vi "_r2aio_16bit_8in_canopen_master.vi"() -> ()   [LabVIEW 2011]
panel:
  out "ret write_device_object_sdo INT":i16
  out "ret write_pdo_mapping 12":i16
  out "Analogue IN 8":i16
  out "ret read_node_object_dictionary 8":i16
  out "Analogue IN 7":i16
  out "ret read_node_object_dictionary 7":i16
  out "Analogue IN 6":i16
  out "ret read_node_object_dictionary 6":i16
  out "Analogue IN 5":i16
  out "ret read_node_object_dictionary 5":i16
  out "Analogue IN 4":i16
  out "ret read_node_object_dictionary 4":i16
  out "Analogue IN 3":i16
  out "ret read_node_object_dictionary 3":i16
  out "Analogue IN 2":i16
  out "ret read_node_object_dictionary 2":i16
  out "Analogue IN 1":i16
  out "ret write_pdo_mapping 11":i16
  out "ret write_pdo_mapping 10":i16
  out "ret write_pdo_mapping 9":i16
  out "ret write_pdo_mapping 8":i16
  out "ret write_pdo_mapping 7":i16
  out "ret write_pdo_mapping 6":i16
  out "ret write_pdo_mapping 5":i16
  out "ret write_pdo_mapping 4":i16
  out "ret write_pdo_mapping 2":i16
  out "ret add_node_object_dictionary 6401-8":i16
  out "ret add_node_object_dictionary 6401-7":i16
  out "ret add_node_object_dictionary 6401-6":i16
  out "ret add_node_object_dictionary 6401-5":i16
  out "ret add_node_object_dictionary 6401-4":i16
  out "ret add_node_object_dictionary 6401-3":i16
  out "ret add_node_object_dictionary 6401-2":i16
  out "datasize":u32
  out "Manufacturer software ver":string
  out "ret read_device_object_sdo 3":i16
  out "datasize":u32
  out "Manufacturer hardware ver":string
  out "ret read_device_object_sdo 2":i16
  out "datasize":u32
  out "Manufacturer dev name":string
  out "ret read_device_object_sdo 1":i16
  out "ret read_node_object_dictionary 1":i16
  in  "stop monitor":bool
  out "ret write_master_hbt":i16
  out "ret stop_can_master":i16
  out "ret write_pdo_mapping 3":i16
  out "ret write_pdo_mapping 1":i16
  out "ret add_node_object_dictionary 6401-1":i16
  out "ret write_device_object_sdo HBT":i16
  in  "slave node":u8
  in  "baudrate":T1(ring)
  in  "net":u8
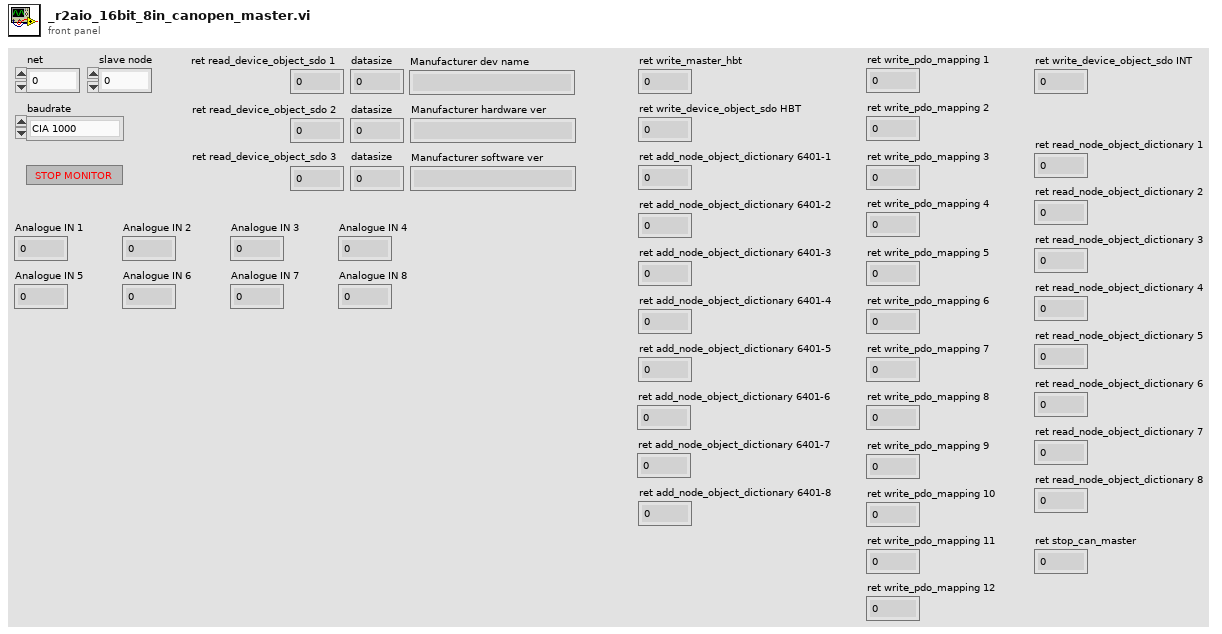
[diagram p1: front panel]
types:
  T1 = enum8{"CIA 1000", "CIA 800", "CIA 500", "CIA 250", "CIA 125", "CIA 100", "CIA 50", "CIA 20", "CIA 10", "CIA AUTO"}
diagram:
  n1 = flat-sequence {
    tunnel: ["slave node"] -> w44
    tunnel: w44 -> [w54]
    tunnel: [w54] -> w43
    tunnel: w43 -> [w56]
    tunnel: [w56] -> w46
    tunnel: w46 -> [w63]
    tunnel: [w63] -> w45
    tunnel: w45 -> [w66]
    tunnel: [w66] -> w40
    tunnel: w40 -> [w71]
    tunnel: [w71] -> w39
    tunnel: w39 -> [w76]
    tunnel: [w76] -> w38
    tunnel: w38 -> [w81]
    tunnel: [w81] -> w37
    tunnel: w37 -> [w86]
    tunnel: [w86] -> w36
    tunnel: w36 -> [w91]
    tunnel: [w91] -> w35
    tunnel: w35 -> [w97]
    tunnel: [w97] -> w34
    tunnel: w34 -> [w101]
    tunnel: [w101] -> w9
    tunnel: [w106] -> w42
    tunnel: w9 -> [w106]
    tunnel: [w111] -> w33
    tunnel: w42 -> [w111]
    tunnel: [w108] -> w21
    tunnel: w33 -> [w121]
    tunnel: [w121] -> w22
    tunnel: w21 -> [w119]
    tunnel: [w119] -> w20
    tunnel: [w128] -> w32
    tunnel: [w126] -> w19
    tunnel: w22 -> [w128]
    tunnel: w20 -> [w126]
    tunnel: w32 -> [w135]
    tunnel: [w135] -> w31
    tunnel: w19 -> [w133]
    tunnel: [w133] -> w18
    tunnel: w31 -> [w141]
    tunnel: [w141] -> w30
    tunnel: w18 -> [w140]
    tunnel: [w140] -> w17
    tunnel: w30 -> [w149]
    tunnel: [w149] -> w29
    tunnel: w17 -> [w147]
    tunnel: [w147] -> w16
    tunnel: w29 -> [w155]
    tunnel: [w155] -> w28
    tunnel: w16 -> [w154]
    tunnel: [w154] -> w15
    tunnel: w28 -> [w163]
    tunnel: [w163] -> w27
    tunnel: w15 -> [w161]
    tunnel: [w161] -> w14
    tunnel: w27 -> [w169]
    tunnel: [w169] -> w26
    tunnel: w14 -> [w168]
    tunnel: [w168] -> w13
    tunnel: w26 -> [w176]
    tunnel: [w176] -> w25
    tunnel: w13 -> [w175]
    tunnel: [w175] -> w12
    tunnel: [w184] -> w24
    tunnel: [w182] -> w11
    tunnel: w12 -> [w182]
    tunnel: w25 -> [w184]
    tunnel: w24 -> [w191]
    tunnel: [w191] -> w23
    tunnel: w11 -> [w189]
    tunnel: [w189] -> w10
    tunnel: [w202] -> w41
    tunnel: w10 -> [_]
    tunnel: w23 -> [w202]
    tunnel: [w204] -> w5
    tunnel: w41 -> [w204]
    tunnel: [w212] -> w7
    tunnel: w5 -> [w212]
    tunnel: w7 -> [w214]
    tunnel: [w214] -> w6
    tunnel: w6 -> [w215]
    tunnel: [w215] -> w4
    tunnel: w4 -> [w224]
    tunnel: [w224] -> w3
    tunnel: w3 -> [w225]
    tunnel: [w225] -> w2
    tunnel: w2 -> [w234]
    tunnel: [w234] -> w1
    tunnel: w1 -> [w236]
    tunnel: [w236] -> w8
    tunnel: w8 -> [w237]
    frame #0 {
      # "Start CAN master"
      n2 = call "start_can_master.vi"("br"="baudrate", "net"="net") -> ("return"=w50:i16)  [unwired: 9 in]
      n3 = Not Equal To 0?(x=w50) -> (x != 0?=w49:bool)
      n4 = Stop(stop? (T)=w49) -> ()
    }
    frame #1 {
      w52 = u8 129 items=["CAN_NMT_CS_DUMMY"=0, "CAN_NMT_START_REMOTE_NODE"=1, "CAN_NMT_STOP_REMOTE_NODE"=2, "CAN_NMT_ENTER_PRE_OPERATIONAL"=128, "CAN_NMT_RESET_NODE"=129, "CAN_NMT_RESET_COMMUNICATION"=130]  # NMT spec
      # "NMT Reset node"
      n5 = call "nmt_master_command.vi"("node"="slave node", "cs"=w52) -> ()  [unwired: 10 in]
    }
    frame #2 {
      n6 = Wait (ms)(milliseconds to wait=u32 500) -> ()  [unwired: 1 out]
    }
    frame #3 {
      # "Configure MASTER Heartbeat"
      n7 = call "write_master_hbt.vi"("hbt"=u16 1200, "node"=w56) -> ("return"=→"ret write_master_hbt":i16)  [unwired: 9 in]
    }
    frame #4 {
      # "Configure SLAVE Heartbeat"
      n8 = Build Array(u8 232, u8 3) -> (w59:u8[])
      n9 = call "write_device_object_sdo.vi"("node"=w63, "index"=u16 4119, "subind"=u8 0, "data"=w59, "datasize"=u32 2) -> ("return"=→"ret write_device_object_sdo HBT":i16)  [unwired: 10 in]
    }
    frame #5 {
      w68 = u16 3 items=["CAN_DEFTYPE_BOOLEAN"=1, "CAN_DEFTYPE_INTEGER8"=2, "CAN_DEFTYPE_INTEGER16"=3, "CAN_DEFTYPE_INTEGER32"=4, "CAN_DEFTYPE_UNSIGNED8"=5, "CAN_DEFTYPE_UNSIGNED16"=6, "CAN_DEFTYPE_UNSIGNED32"=7, "CAN_DEFTYPE_REAL32"=8, "CAN_DEFTYPE_VISIBLE_STRING"=9, "CAN_DEFTYPE_OCTET_STRING"=10, "CAN_DEFTYPE_UNICODE_STRING"=11, "CAN_DEFTYPE_TIME_OF_DAY"=12, "CAN_DEFTYPE_TIME_DIFFERENCE"=13, "CAN_DEFTYPE_DOMAIN"=15, "CAN_DEFTYPE_INTEGER24"=16, "CAN_DEFTYPE_REAL64"=17, "CAN_DEFTYPE_INTEGER40"=18, "CAN_DEFTYPE_INTEGER48"=19, "CAN_DEFTYPE_INTEGER56"=20, "CAN_DEFTYPE_INTEGER64"=21, "CAN_DEFTYPE_UNSIGNED24"=22, "CAN_DEFTYPE_UNSIGNED40"=24, "CAN_DEFTYPE_UNSIGNED48"=25, "CAN_DEFTYPE_UNSIGNED56"=26, "CAN_DEFTYPE_UNSIGNED64"=27]  # Data type spec
      # "Add Read Analogue input 1 object to MASTER dictionary"
      n10 = call "add_node_object_dictionary.vi"("type"=w68, "subind"=u8 1, "index"=u16 25601, "node"=w66) -> ("return"=→"ret add_node_object_dictionary 6401-1":i16)  [unwired: 7 in]
    }
    frame #6 {
      w73 = u16 3 items=["CAN_DEFTYPE_BOOLEAN"=1, "CAN_DEFTYPE_INTEGER8"=2, "CAN_DEFTYPE_INTEGER16"=3, "CAN_DEFTYPE_INTEGER32"=4, "CAN_DEFTYPE_UNSIGNED8"=5, "CAN_DEFTYPE_UNSIGNED16"=6, "CAN_DEFTYPE_UNSIGNED32"=7, "CAN_DEFTYPE_REAL32"=8, "CAN_DEFTYPE_VISIBLE_STRING"=9, "CAN_DEFTYPE_OCTET_STRING"=10, "CAN_DEFTYPE_UNICODE_STRING"=11, "CAN_DEFTYPE_TIME_OF_DAY"=12, "CAN_DEFTYPE_TIME_DIFFERENCE"=13, "CAN_DEFTYPE_DOMAIN"=15, "CAN_DEFTYPE_INTEGER24"=16, "CAN_DEFTYPE_REAL64"=17, "CAN_DEFTYPE_INTEGER40"=18, "CAN_DEFTYPE_INTEGER48"=19, "CAN_DEFTYPE_INTEGER56"=20, "CAN_DEFTYPE_INTEGER64"=21, "CAN_DEFTYPE_UNSIGNED24"=22, "CAN_DEFTYPE_UNSIGNED40"=24, "CAN_DEFTYPE_UNSIGNED48"=25, "CAN_DEFTYPE_UNSIGNED56"=26, "CAN_DEFTYPE_UNSIGNED64"=27]  # Data type spec
      # "Add Read Analogue input 2 object to MASTER dictionary"
      n11 = call "add_node_object_dictionary.vi"("type"=w73, "subind"=u8 2, "index"=u16 25601, "node"=w71) -> ("return"=→"ret add_node_object_dictionary 6401-2":i16)  [unwired: 7 in]
    }
    frame #7 {
      w78 = u16 3 items=["CAN_DEFTYPE_BOOLEAN"=1, "CAN_DEFTYPE_INTEGER8"=2, "CAN_DEFTYPE_INTEGER16"=3, "CAN_DEFTYPE_INTEGER32"=4, "CAN_DEFTYPE_UNSIGNED8"=5, "CAN_DEFTYPE_UNSIGNED16"=6, "CAN_DEFTYPE_UNSIGNED32"=7, "CAN_DEFTYPE_REAL32"=8, "CAN_DEFTYPE_VISIBLE_STRING"=9, "CAN_DEFTYPE_OCTET_STRING"=10, "CAN_DEFTYPE_UNICODE_STRING"=11, "CAN_DEFTYPE_TIME_OF_DAY"=12, "CAN_DEFTYPE_TIME_DIFFERENCE"=13, "CAN_DEFTYPE_DOMAIN"=15, "CAN_DEFTYPE_INTEGER24"=16, "CAN_DEFTYPE_REAL64"=17, "CAN_DEFTYPE_INTEGER40"=18, "CAN_DEFTYPE_INTEGER48"=19, "CAN_DEFTYPE_INTEGER56"=20, "CAN_DEFTYPE_INTEGER64"=21, "CAN_DEFTYPE_UNSIGNED24"=22, "CAN_DEFTYPE_UNSIGNED40"=24, "CAN_DEFTYPE_UNSIGNED48"=25, "CAN_DEFTYPE_UNSIGNED56"=26, "CAN_DEFTYPE_UNSIGNED64"=27]  # Data type spec
      # "Add Read Analogue input 3 object to MASTER dictionary"
      n12 = call "add_node_object_dictionary.vi"("type"=w78, "subind"=u8 3, "index"=u16 25601, "node"=w76) -> ("return"=→"ret add_node_object_dictionary 6401-3":i16)  [unwired: 7 in]
    }
    frame #8 {
      w83 = u16 3 items=["CAN_DEFTYPE_BOOLEAN"=1, "CAN_DEFTYPE_INTEGER8"=2, "CAN_DEFTYPE_INTEGER16"=3, "CAN_DEFTYPE_INTEGER32"=4, "CAN_DEFTYPE_UNSIGNED8"=5, "CAN_DEFTYPE_UNSIGNED16"=6, "CAN_DEFTYPE_UNSIGNED32"=7, "CAN_DEFTYPE_REAL32"=8, "CAN_DEFTYPE_VISIBLE_STRING"=9, "CAN_DEFTYPE_OCTET_STRING"=10, "CAN_DEFTYPE_UNICODE_STRING"=11, "CAN_DEFTYPE_TIME_OF_DAY"=12, "CAN_DEFTYPE_TIME_DIFFERENCE"=13, "CAN_DEFTYPE_DOMAIN"=15, "CAN_DEFTYPE_INTEGER24"=16, "CAN_DEFTYPE_REAL64"=17, "CAN_DEFTYPE_INTEGER40"=18, "CAN_DEFTYPE_INTEGER48"=19, "CAN_DEFTYPE_INTEGER56"=20, "CAN_DEFTYPE_INTEGER64"=21, "CAN_DEFTYPE_UNSIGNED24"=22, "CAN_DEFTYPE_UNSIGNED40"=24, "CAN_DEFTYPE_UNSIGNED48"=25, "CAN_DEFTYPE_UNSIGNED56"=26, "CAN_DEFTYPE_UNSIGNED64"=27]  # Data type spec
      # "Add Read Analogue input 4 object to MASTER dictionary"
      n13 = call "add_node_object_dictionary.vi"("type"=w83, "subind"=u8 4, "index"=u16 25601, "node"=w81) -> ("return"=→"ret add_node_object_dictionary 6401-4":i16)  [unwired: 7 in]
    }
    frame #9 {
      w88 = u16 3 items=["CAN_DEFTYPE_BOOLEAN"=1, "CAN_DEFTYPE_INTEGER8"=2, "CAN_DEFTYPE_INTEGER16"=3, "CAN_DEFTYPE_INTEGER32"=4, "CAN_DEFTYPE_UNSIGNED8"=5, "CAN_DEFTYPE_UNSIGNED16"=6, "CAN_DEFTYPE_UNSIGNED32"=7, "CAN_DEFTYPE_REAL32"=8, "CAN_DEFTYPE_VISIBLE_STRING"=9, "CAN_DEFTYPE_OCTET_STRING"=10, "CAN_DEFTYPE_UNICODE_STRING"=11, "CAN_DEFTYPE_TIME_OF_DAY"=12, "CAN_DEFTYPE_TIME_DIFFERENCE"=13, "CAN_DEFTYPE_DOMAIN"=15, "CAN_DEFTYPE_INTEGER24"=16, "CAN_DEFTYPE_REAL64"=17, "CAN_DEFTYPE_INTEGER40"=18, "CAN_DEFTYPE_INTEGER48"=19, "CAN_DEFTYPE_INTEGER56"=20, "CAN_DEFTYPE_INTEGER64"=21, "CAN_DEFTYPE_UNSIGNED24"=22, "CAN_DEFTYPE_UNSIGNED40"=24, "CAN_DEFTYPE_UNSIGNED48"=25, "CAN_DEFTYPE_UNSIGNED56"=26, "CAN_DEFTYPE_UNSIGNED64"=27]  # Data type spec
      # "Add Read Analogue input 5 object to MASTER dictionary"
      n14 = call "add_node_object_dictionary.vi"("type"=w88, "subind"=u8 5, "index"=u16 25601, "node"=w86) -> ("return"=→"ret add_node_object_dictionary 6401-5":i16)  [unwired: 7 in]
    }
    frame #10 {
      w93 = u16 3 items=["CAN_DEFTYPE_BOOLEAN"=1, "CAN_DEFTYPE_INTEGER8"=2, "CAN_DEFTYPE_INTEGER16"=3, "CAN_DEFTYPE_INTEGER32"=4, "CAN_DEFTYPE_UNSIGNED8"=5, "CAN_DEFTYPE_UNSIGNED16"=6, "CAN_DEFTYPE_UNSIGNED32"=7, "CAN_DEFTYPE_REAL32"=8, "CAN_DEFTYPE_VISIBLE_STRING"=9, "CAN_DEFTYPE_OCTET_STRING"=10, "CAN_DEFTYPE_UNICODE_STRING"=11, "CAN_DEFTYPE_TIME_OF_DAY"=12, "CAN_DEFTYPE_TIME_DIFFERENCE"=13, "CAN_DEFTYPE_DOMAIN"=15, "CAN_DEFTYPE_INTEGER24"=16, "CAN_DEFTYPE_REAL64"=17, "CAN_DEFTYPE_INTEGER40"=18, "CAN_DEFTYPE_INTEGER48"=19, "CAN_DEFTYPE_INTEGER56"=20, "CAN_DEFTYPE_INTEGER64"=21, "CAN_DEFTYPE_UNSIGNED24"=22, "CAN_DEFTYPE_UNSIGNED40"=24, "CAN_DEFTYPE_UNSIGNED48"=25, "CAN_DEFTYPE_UNSIGNED56"=26, "CAN_DEFTYPE_UNSIGNED64"=27]  # Data type spec
      # "Add Read Analogue input 6 object to MASTER dictionary"
      n15 = call "add_node_object_dictionary.vi"("type"=w93, "subind"=u8 6, "index"=u16 25601, "node"=w91) -> ("return"=→"ret add_node_object_dictionary 6401-6":i16)  [unwired: 7 in]
    }
    frame #11 {
      w96 = u16 3 items=["CAN_DEFTYPE_BOOLEAN"=1, "CAN_DEFTYPE_INTEGER8"=2, "CAN_DEFTYPE_INTEGER16"=3, "CAN_DEFTYPE_INTEGER32"=4, "CAN_DEFTYPE_UNSIGNED8"=5, "CAN_DEFTYPE_UNSIGNED16"=6, "CAN_DEFTYPE_UNSIGNED32"=7, "CAN_DEFTYPE_REAL32"=8, "CAN_DEFTYPE_VISIBLE_STRING"=9, "CAN_DEFTYPE_OCTET_STRING"=10, "CAN_DEFTYPE_UNICODE_STRING"=11, "CAN_DEFTYPE_TIME_OF_DAY"=12, "CAN_DEFTYPE_TIME_DIFFERENCE"=13, "CAN_DEFTYPE_DOMAIN"=15, "CAN_DEFTYPE_INTEGER24"=16, "CAN_DEFTYPE_REAL64"=17, "CAN_DEFTYPE_INTEGER40"=18, "CAN_DEFTYPE_INTEGER48"=19, "CAN_DEFTYPE_INTEGER56"=20, "CAN_DEFTYPE_INTEGER64"=21, "CAN_DEFTYPE_UNSIGNED24"=22, "CAN_DEFTYPE_UNSIGNED40"=24, "CAN_DEFTYPE_UNSIGNED48"=25, "CAN_DEFTYPE_UNSIGNED56"=26, "CAN_DEFTYPE_UNSIGNED64"=27]  # Data type spec
      # "Add Read Analogue input 7 object to MASTER dictionary"
      n16 = call "add_node_object_dictionary.vi"("type"=w96, "subind"=u8 7, "index"=u16 25601, "node"=w97) -> ("return"=→"ret add_node_object_dictionary 6401-7":i16)  [unwired: 7 in]
    }
    frame #12 {
      w103 = u16 3 items=["CAN_DEFTYPE_BOOLEAN"=1, "CAN_DEFTYPE_INTEGER8"=2, "CAN_DEFTYPE_INTEGER16"=3, "CAN_DEFTYPE_INTEGER32"=4, "CAN_DEFTYPE_UNSIGNED8"=5, "CAN_DEFTYPE_UNSIGNED16"=6, "CAN_DEFTYPE_UNSIGNED32"=7, "CAN_DEFTYPE_REAL32"=8, "CAN_DEFTYPE_VISIBLE_STRING"=9, "CAN_DEFTYPE_OCTET_STRING"=10, "CAN_DEFTYPE_UNICODE_STRING"=11, "CAN_DEFTYPE_TIME_OF_DAY"=12, "CAN_DEFTYPE_TIME_DIFFERENCE"=13, "CAN_DEFTYPE_DOMAIN"=15, "CAN_DEFTYPE_INTEGER24"=16, "CAN_DEFTYPE_REAL64"=17, "CAN_DEFTYPE_INTEGER40"=18, "CAN_DEFTYPE_INTEGER48"=19, "CAN_DEFTYPE_INTEGER56"=20, "CAN_DEFTYPE_INTEGER64"=21, "CAN_DEFTYPE_UNSIGNED24"=22, "CAN_DEFTYPE_UNSIGNED40"=24, "CAN_DEFTYPE_UNSIGNED48"=25, "CAN_DEFTYPE_UNSIGNED56"=26, "CAN_DEFTYPE_UNSIGNED64"=27]  # Data type spec
      # "Add Read Analogue input 8 object to MASTER dictionary"
      n17 = call "add_node_object_dictionary.vi"("type"=w103, "subind"=u8 8, "index"=u16 25601, "node"=w101) -> ("return"=→"ret add_node_object_dictionary 6401-8":i16)  [unwired: 7 in]
    }
    frame #13 {
      w107 = u8 1 items=["CAN_NMT_CS_DUMMY"=0, "CAN_NMT_START_REMOTE_NODE"=1, "CAN_NMT_STOP_REMOTE_NODE"=2, "CAN_NMT_ENTER_PRE_OPERATIONAL"=128, "CAN_NMT_RESET_NODE"=129, "CAN_NMT_RESET_COMMUNICATION"=130]  # NMT spec
      # "NMT Start remote node"
      n18 = call "nmt_master_command.vi"("node"=w106, "cs"=w107) -> ()  [unwired: 10 in]
    }
    frame #14 {
      # "Disable RPDO2 mapping"
      n19 = Subtract(x=w111, y=u8 1) -> (x-y=w110:u8)
      n20 = Multiply(x=w110, y=u8 4) -> (x*y=w109:u8)
      n21 = To Unsigned Word Integer(number=w109) -> (unsigned 16bit integer=w108:u16)
      n22 = Add(x=w108, y=u16 5633) -> (x+y=w114:u16)
      n23 = call "write_pdo_mapping.vi"("data"=u32 0, "subind"=u8 0, "index"=w114) -> ("return"=→"ret write_pdo_mapping 1":i16)  [unwired: 8 in]
    }
    frame #15 {
      # "Disable RPDO3 mapping"
      n24 = Add(x=w119, y=u16 5634) -> (x+y=w120:u16)
      n25 = call "write_pdo_mapping.vi"("data"=u32 0, "subind"=u8 0, "index"=w120) -> ("return"=→"ret write_pdo_mapping 2":i16)  [unwired: 8 in]
    }
    frame #16 {
      # "Map Read Analogue Input 1 RPDO2"
      n26 = Add(x=w126, y=u16 5633) -> (x+y=w127:u16)
      n27 = call "write_pdo_mapping.vi"("data"=u32 1677787408, "subind"=u8 1, "index"=w127) -> ("return"=→"ret write_pdo_mapping 3":i16)  [unwired: 8 in]
    }
    frame #17 {
      # "Map Read Analogue Input 2 RPDO2"
      n28 = Add(x=w133, y=u16 5633) -> (x+y=w134:u16)
      n29 = call "write_pdo_mapping.vi"("data"=u32 1677787664, "subind"=u8 2, "index"=w134) -> ("return"=→"ret write_pdo_mapping 4":i16)  [unwired: 8 in]
    }
    frame #18 {
      # "Map Read Analogue Input 3 RPDO2"
      n30 = Add(x=w140, y=u16 5633) -> (x+y=w143:u16)
      n31 = call "write_pdo_mapping.vi"("data"=u32 1677787920, "subind"=u8 3, "index"=w143) -> ("return"=→"ret write_pdo_mapping 5":i16)  [unwired: 8 in]
    }
    frame #19 {
      # "Map Read Analogue Input 4 RPDO2"
      n32 = Add(x=w147, y=u16 5633) -> (x+y=w148:u16)
      n33 = call "write_pdo_mapping.vi"("data"=u32 1677788176, "subind"=u8 4, "index"=w148) -> ("return"=→"ret write_pdo_mapping 6":i16)  [unwired: 8 in]
    }
    frame #20 {
      # "Map Read Analogue Input 5 RPDO3"
      n34 = Add(x=w154, y=u16 5634) -> (x+y=w156:u16)
      n35 = call "write_pdo_mapping.vi"("data"=u32 1677788432, "subind"=u8 1, "index"=w156) -> ("return"=→"ret write_pdo_mapping 7":i16)  [unwired: 8 in]
    }
    frame #21 {
      # "Map Read Analogue Input 6 RPDO3"
      n36 = Add(x=w161, y=u16 5634) -> (x+y=w162:u16)
      n37 = call "write_pdo_mapping.vi"("data"=u32 1677788688, "subind"=u8 2, "index"=w162) -> ("return"=→"ret write_pdo_mapping 8":i16)  [unwired: 8 in]
    }
    frame #22 {
      # "Map Read Analogue Input 7 RPDO3"
      n38 = Add(x=w168, y=u16 5634) -> (x+y=w171:u16)
      n39 = call "write_pdo_mapping.vi"("data"=u32 1677788944, "subind"=u8 3, "index"=w171) -> ("return"=→"ret write_pdo_mapping 9":i16)  [unwired: 8 in]
    }
    frame #23 {
      # "Map Read Analogue Input 8 RPDO3"
      n40 = Add(x=w175, y=u16 5634) -> (x+y=w178:u16)
      n41 = call "write_pdo_mapping.vi"("data"=u32 1677789200, "subind"=u8 4, "index"=w178) -> ("return"=→"ret write_pdo_mapping 10":i16)  [unwired: 8 in]
    }
    frame #24 {
      # "Enable RPDO2 mapping"
      n42 = Add(x=w182, y=u16 5633) -> (x+y=w183:u16)
      n43 = call "write_pdo_mapping.vi"("data"=u32 4, "subind"=u8 0, "index"=w183) -> ("return"=→"ret write_pdo_mapping 11":i16)  [unwired: 8 in]
    }
    frame #25 {
      # "Enable RPDO3 mapping"
      n44 = Add(x=w189, y=u16 5634) -> (x+y=w190:u16)
      n45 = call "write_pdo_mapping.vi"("data"=u32 4, "subind"=u8 0, "index"=w190) -> ("return"=→"ret write_pdo_mapping 12":i16)  [unwired: 8 in]
    }
    frame #26 {
      # "Enable GLOBAL interrupts"
      n46 = Build Array(u8 1) -> (w198:u8[])
      n47 = call "write_device_object_sdo.vi"("node"=w202, "index"=u16 25635, "subind"=u8 0, "data"=w198, "datasize"=u32 1) -> ("return"=→"ret write_device_object_sdo INT":i16)  [unwired: 10 in]
    }
    frame #27 {
      n48 = Wait (ms)(milliseconds to wait=u32 500) -> ()  [unwired: 1 out]
    }
    frame #28 {
      # "Read Manufacturer Device Name"
      n49 = call "read_device_object_sdo.vi"("node"=w212, "index"=u16 4104, "subind"=u8 0, "datasize"=u32 128) -> ("return"=→"ret read_device_object_sdo 1":i16, "data"=w207:u8[], "datasize"=→"datasize":u32)  [unwired: 9 in]
      n50 = Byte Array To String(unsigned byte array=w207) -> (string=→"Manufacturer dev name":string)
    }
    frame #29 {
      n51 = Wait (ms)(milliseconds to wait=u32 500) -> ()  [unwired: 1 out]
    }
    frame #30 {
      # "Read Manufacturer Hardware Version"
      n52 = call "read_device_object_sdo.vi"("node"=w215, "index"=u16 4105, "subind"=u8 0, "datasize"=u32 128) -> ("return"=→"ret read_device_object_sdo 2":i16, "data"=w218:u8[], "datasize"=→"datasize":u32)  [unwired: 9 in]
      n53 = Byte Array To String(unsigned byte array=w218) -> (string=→"Manufacturer hardware ver":string)
    }
    frame #31 {
      n54 = Wait (ms)(milliseconds to wait=u32 500) -> ()  [unwired: 1 out]
    }
    frame #32 {
      # "Read Manufacturer Software Version"
      n55 = call "read_device_object_sdo.vi"("node"=w225, "index"=u16 4106, "subind"=u8 0, "datasize"=u32 128) -> ("return"=→"ret read_device_object_sdo 3":i16, "data"=w228:u8[], "datasize"=→"datasize":u32)  [unwired: 9 in]
      n56 = Byte Array To String(unsigned byte array=w228) -> (string=→"Manufacturer software ver":string)
    }
    frame #33 {
      n57 = Wait (ms)(milliseconds to wait=u32 500) -> ()  [unwired: 1 out]
    }
    frame #34 {
      w235 = u8 1 items=["NOT_VALID", "VALID"]  # State
      # "Set all PDOs valid"
      n58 = call "set_all_pdos_state.vi"("state"=w235) -> ()  [unwired: 11 in]
    }
    frame #35 {
      # "Monitor"
      n59 = while {
        tunnel: w237 -> [w238]
        stop <- "stop monitor" stop-if-true
        n60 = call "read_node_object_dictionary.vi"("node"=w238, "index"=u16 25601, "subind"=u8 1) -> ("return"=→"ret read_node_object_dictionary 1":i16, "num"=w275:u64)  [unwired: 10 in, 1 out]
        n61 = To Word Integer(number=w275) -> (16bit integer=→"Analogue IN 1":i16)
        n62 = call "read_node_object_dictionary.vi"("node"=w238, "index"=u16 25601, "subind"=u8 2) -> ("return"=→"ret read_node_object_dictionary 2":i16, "num"=w270:u64)  [unwired: 10 in, 1 out]
        n63 = To Word Integer(number=w270) -> (16bit integer=→"Analogue IN 2":i16)
        n64 = call "read_node_object_dictionary.vi"("node"=w238, "index"=u16 25601, "subind"=u8 3) -> ("return"=→"ret read_node_object_dictionary 3":i16, "num"=w265:u64)  [unwired: 10 in, 1 out]
        n65 = To Word Integer(number=w265) -> (16bit integer=→"Analogue IN 3":i16)
        n66 = call "read_node_object_dictionary.vi"("node"=w238, "index"=u16 25601, "subind"=u8 4) -> ("return"=→"ret read_node_object_dictionary 4":i16, "num"=w260:u64)  [unwired: 10 in, 1 out]
        n67 = To Word Integer(number=w260) -> (16bit integer=→"Analogue IN 4":i16)
        n68 = call "read_node_object_dictionary.vi"("node"=w238, "index"=u16 25601, "subind"=u8 5) -> ("return"=→"ret read_node_object_dictionary 5":i16, "num"=w255:u64)  [unwired: 10 in, 1 out]
        n69 = To Word Integer(number=w255) -> (16bit integer=→"Analogue IN 5":i16)
        n70 = call "read_node_object_dictionary.vi"("node"=w238, "index"=u16 25601, "subind"=u8 6) -> ("return"=→"ret read_node_object_dictionary 6":i16, "num"=w250:u64)  [unwired: 10 in, 1 out]
        n71 = To Word Integer(number=w250) -> (16bit integer=→"Analogue IN 6":i16)
        n72 = call "read_node_object_dictionary.vi"("node"=w238, "index"=u16 25601, "subind"=u8 7) -> ("return"=→"ret read_node_object_dictionary 7":i16, "num"=w245:u64)  [unwired: 10 in, 1 out]
        n73 = To Word Integer(number=w245) -> (16bit integer=→"Analogue IN 7":i16)
        n74 = call "read_node_object_dictionary.vi"("node"=w238, "index"=u16 25601, "subind"=u8 8) -> ("return"=→"ret read_node_object_dictionary 8":i16, "num"=w240:u64)  [unwired: 10 in, 1 out]
        n75 = To Word Integer(number=w240) -> (16bit integer=→"Analogue IN 8":i16)
      }
    }
    frame #36 {
      # "Stop CAN master"
      n76 = call "stop_can_master.vi"() -> ("return"=→"ret stop_can_master":i16)  [unwired: 11 in]
    }
  }
